vi "Camera Tester.vi"() -> ()   [LabVIEW 2024]
doc: "Use this template to build a user interface event handler design pattern. Use this pattern for dialog boxes and other user interfaces. You also can create and execute user-defined events that the VI can handle the same way as user interface events."
uses:
  camera.ctl
  camera driver.ctl
  <vilib>/event_ctls.llb/lveventtype.ctl
  Vision.lvlib
  <vilib>/Utility/error.llb/DialogType.ctl
panel:
  in  "refresh cameras":bool
  in  "Enable imaqdx":bool
  out "String":string
  in  "info tabs":enum32{"Modes", "Properties"}(tab)
  out "Available modes":string
  out "properties":string
  out "Image":T1(plugin-control)
  in  "Save Config":bool
  in  "Open Camera":bool
  out "Camera Selection":T2[](array[typedef])
  in  "Close Camera":bool
  # "Scroll to select camera. If your camera does not show up, try enabling\nimaqdx and refreshing the list."
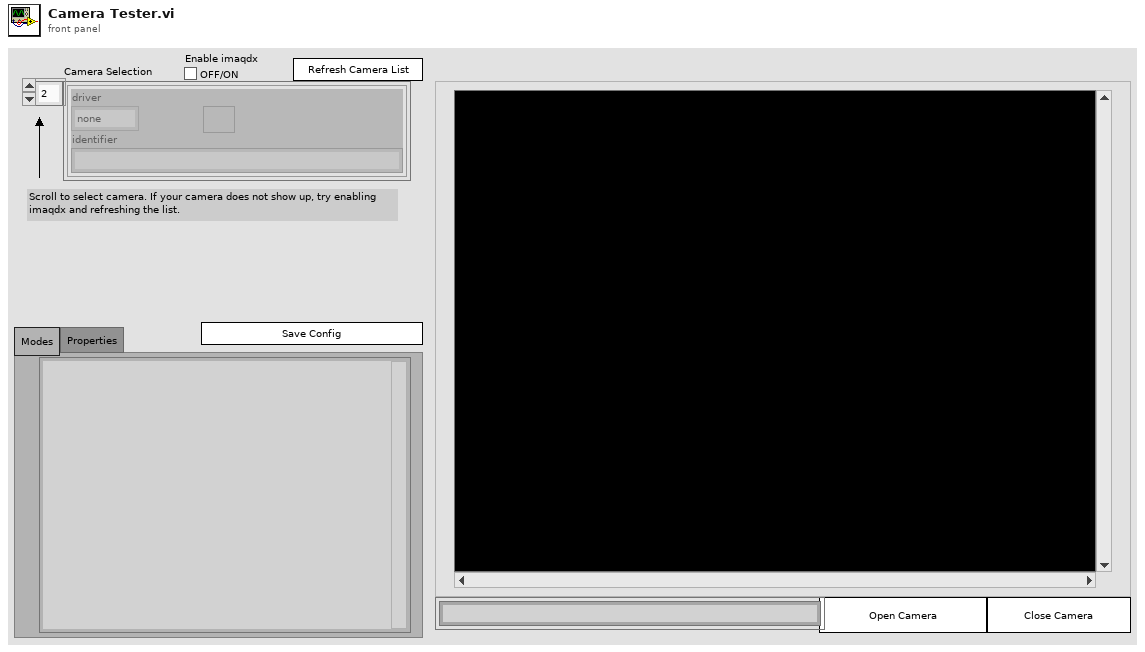
[diagram p1: front panel]
types:
  T1 = typedef "IMAQ Image.ctl" = refnum<image>
  T2 = typedef "Vision.lvlib/camera.ctl" = cluster{"camera reference":variant, "driver":T3, "identifier":string}
  T3 = typedef "Vision.lvlib/camera driver.ctl" = enum16{"none", "wmf", "imaqdx", "peak"}
  T4 = enum8{"Enabled", "Disabled", "Disabled and Grayed Out"}
  T5 = typedef "lveventtype.ctl" = enum32{"Null", "Timeout", "Annotation Menu Selection", "Annotation Menu Selection?", "App Instance Close", "App Instance Close?", "Autoscale Range Change", "Bookmark Info Change", "Cell Edit", "Cell Edit?", "Cursor Grab", "Cursor Grab?", "Cursor Menu Selection", "Cursor Menu Selection?", "Cursor Move", "Cursor Release", "Data Change", "Direction Change", "Display State Change", "Drag Ended", "Drag Enter", "Drag Leave", "Drag Over", "Drag Source Update", "Drag Starting", "Drag Starting?", "Drop", "Exec State Change", "Key Down", "Key Down?", "Key Repeat", "Key Repeat?", "Key Up", "Listbox Double Click", "Menu Activation?", "Menu Selection (App)", "Menu Selection? (App)", "Menu Selection (User)", "Mouse Down", "Mouse Down?", "Mouse Enter", "Mouse Leave", "Mouse Move", "Mouse Up", "Mouse Wheel", "NI Security User Change (App)", "Pane Size", "Panel Close", "Panel Close?", "Panel Resize", "Plot Attribute Change", "Scale Range Change", "Shortcut Menu Activation?", "Shortcut Menu Selection (App)", "Shortcut Menu Selection? (App)", "Shortcut Menu Selection (User)", "Tree Double Click", "Tree Drag", "Tree Drag?", "Tree Drop", "Tree Drop?", "Tree Item Close", "Tree Item Close?", "Tree Item Open", "Tree Item Open?", "User Event", "Value Change"}
  T6 = typedef "DialogType.ctl" = u16
  T7 = typedef "camera mode.ctl" = cluster{"id":i32, "width":i32, "height":i32, "framerate":sgl}
  T8 = cluster{"prop name":string, "value":sgl, "auto":bool}[]
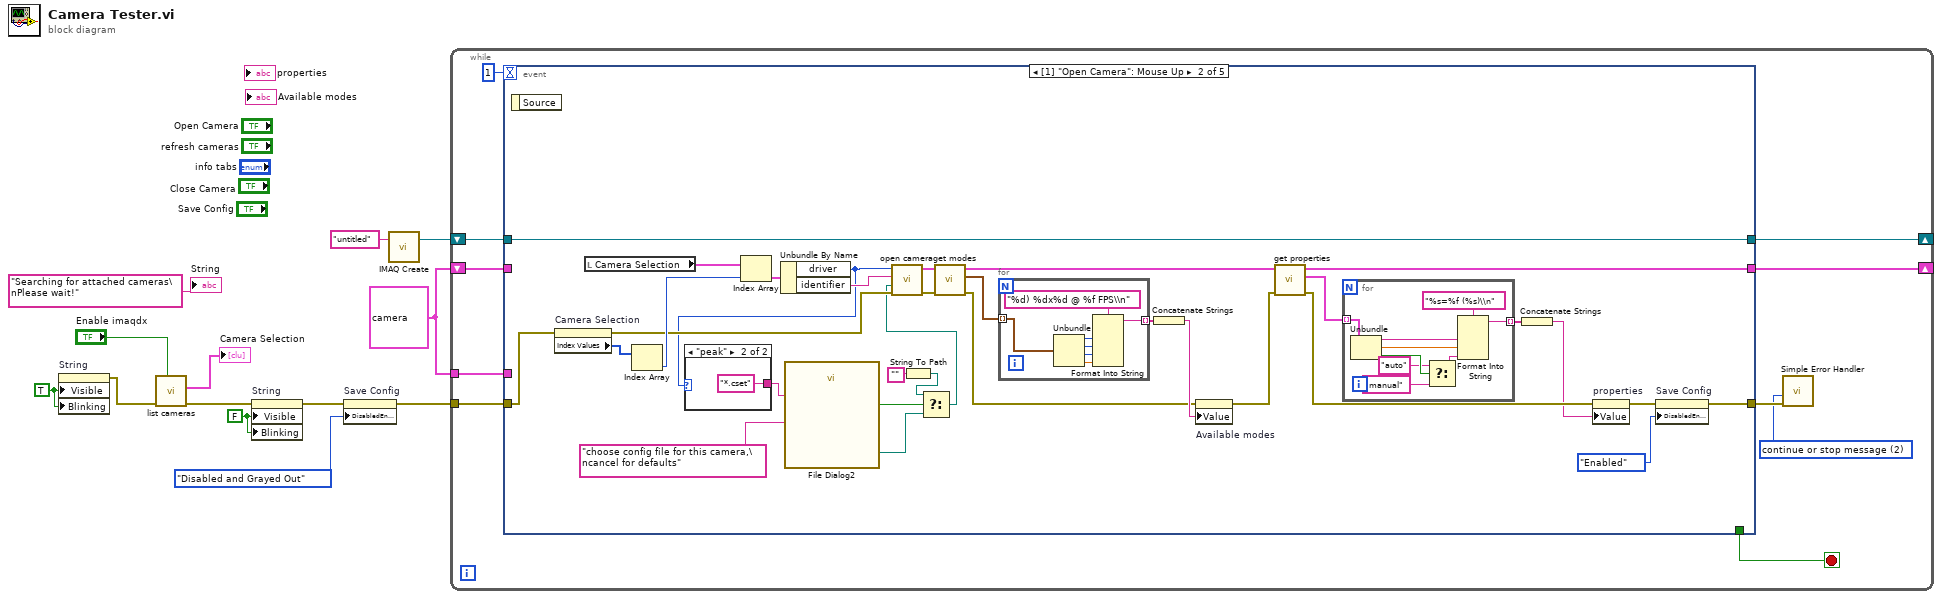
[diagram p0: block diagram]
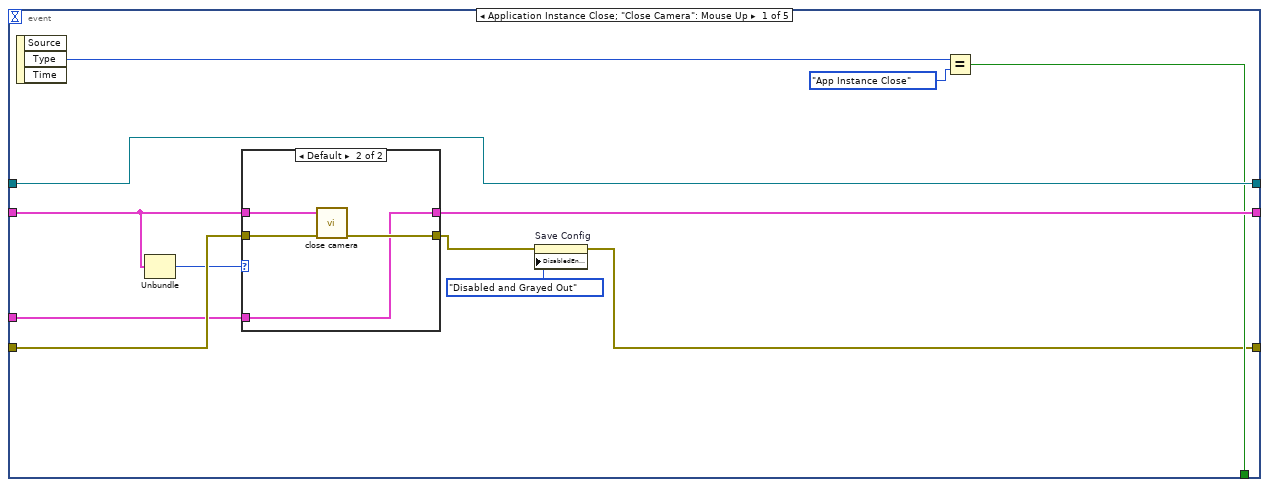
[diagram p2: hidden frame]
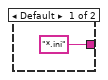
[diagram p4: hidden frame]
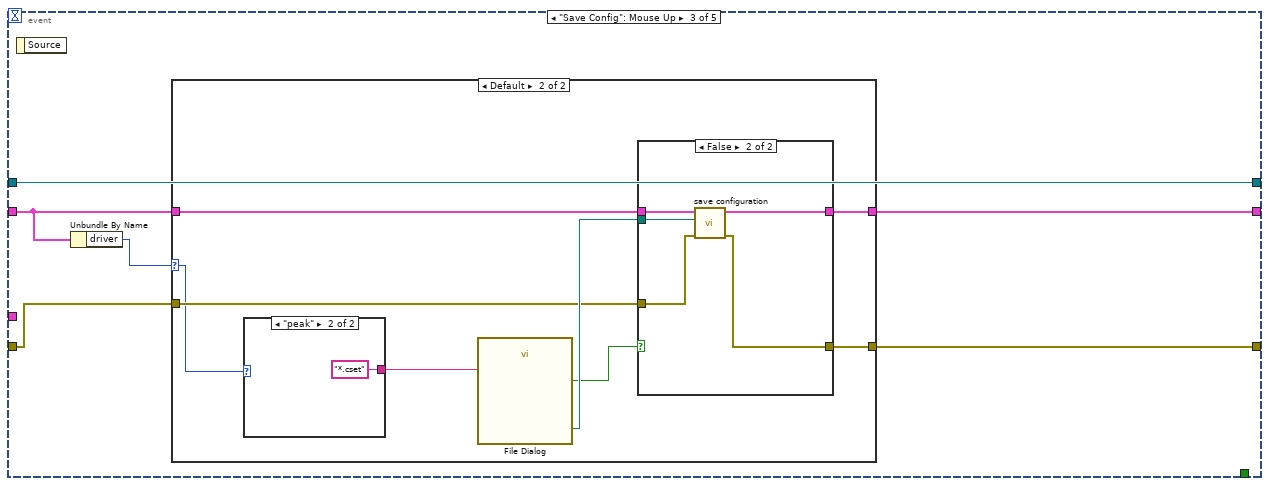
[diagram p5: hidden frame]
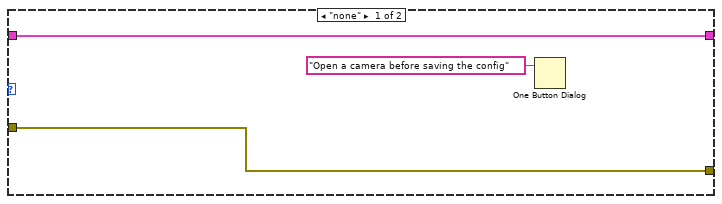
[diagram p6: hidden frame]
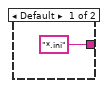
[diagram p7: hidden frame]
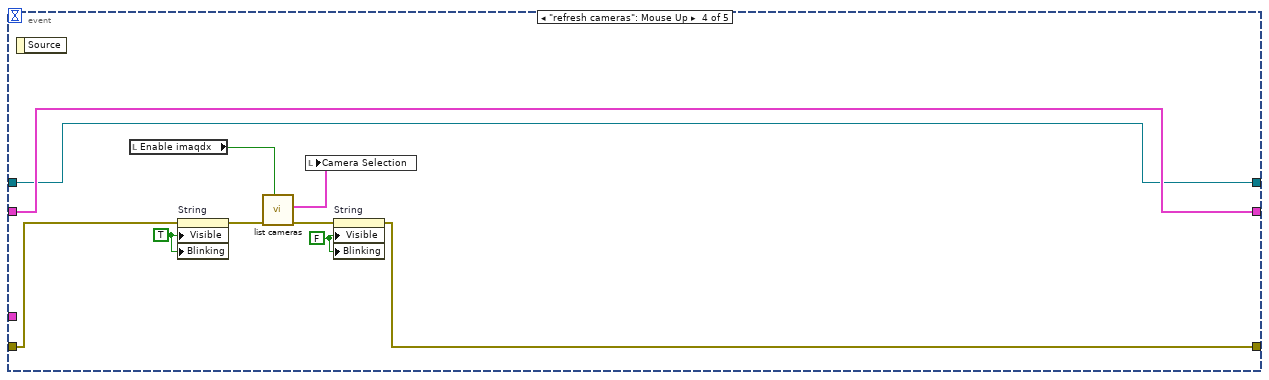
[diagram p9: hidden frame]
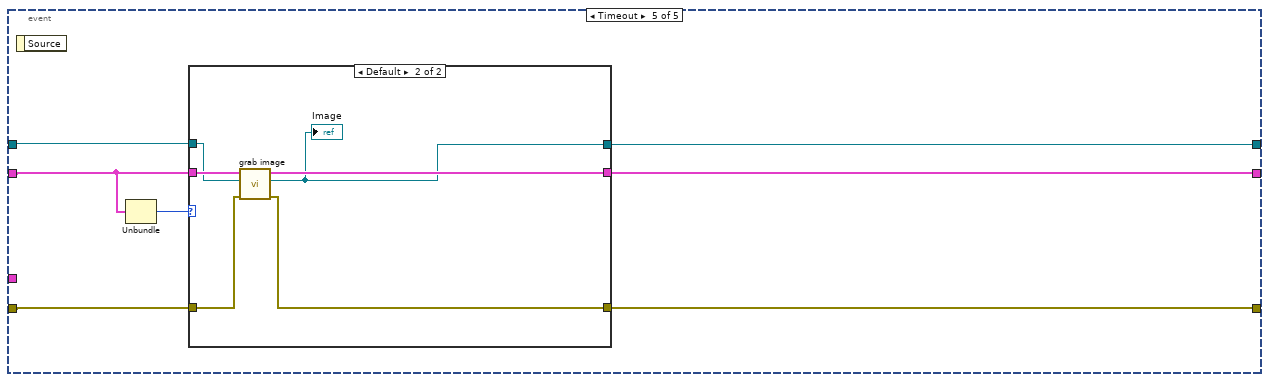
[diagram p10: hidden frame]
diagram:
  w6 = FALSE ("Visible")
  w8 = TRUE ("Visible")
  w4 = T2 {"camera reference"=variant, "driver"=enum."none", "identifier"=""} ("Camera")
  n1 = property on="String" class="Str"("Visible"=w8, "Blinking"=w8) -> (error out=w9:errorcluster)  [unwired: 2 in, 1 out]
  n2 = call "list cameras.vi"("Enable imaqdx"="Enable imaqdx", "error in (no error)"=w9) -> ("error out"=w7:errorcluster, "Cameras"=→"Camera Selection":T2[])  [unwired: 8 in]
  n3 = property on="String" class="Str"(error in=w7, "Visible"=w6, "Blinking"=w6) -> (error out=w2:errorcluster)  [unwired: 1 in, 1 out]
  n4 = property on="Save Config" class="Bool (strict)"(error in=w2, "DisabledEnum"=T4."Disabled and Grayed Out" ("Disabled")) -> (error out=w1:errorcluster)  [unwired: 1 in, 1 out]
  n5 = call "IMAQ Create"("Image Name"="untitled") -> ("New Image"=w12:T1)  [unwired: 4 in, 1 out]
  n6 = while {
    tunnel: w1 -> [w21]
    shift-right: [w19] -> _
    shift-left: w4 -> [w18]
    shift-right: [w17] -> _
    shift-left: w12 -> [w22]
    tunnel: w4 -> [w16]
    stop <- w15 stop-if-true
    w14 = T6 2 items=["no dialog", "OK message", "continue or stop message", "OK message + warnings", "continue/stop + warnings"] ("type of dialog (OK msg:1)")
    n7 = event shown="[1] \"Open Camera\": Mouse Up" {
      selector: _ -> [_ _ _ _ _]
      dyn-events: _ -> [_ _ _ _ _]
      timeout: 1 -> [_ _ _ _ _]
      tunnel: [w28 _ _ _ _] -> w15
      tunnel: w22 -> [w31 w65 w97 w118 w132]
      tunnel: w21 -> [w35 w70 w95 w127 w131]
      tunnel: [w25 w42 w96 w120 w130] -> w20
      tunnel: [w31 w65 w97 w118 w128] -> w17
      tunnel: [w32 w56 w94 w119 w129] -> w19
      tunnel: w18 -> [w34 _ w93 w119 w133]
      tunnel: w16 -> [w27 _ _ _ _]
      event Application Instance Close; "Close Camera": Mouse Up {
        n8 = event-data() -> ("Type"=w30:T5)  [unwired: 1 in, 2 out]
        n9 = Unbundle(w34) -> ("driver"=w33:T3)  [unwired: 2 out]
        n10 = case shown="Default" w33 {
          tunnel: w34 -> [w37 w41]
          tunnel: w35 -> [w36 w40]
          tunnel: [w37 w38] -> w32
          tunnel: [w36 w39] -> w26
          tunnel: w27 -> [_ w38]
          frame "none" {
          }
          frame Default {
            n11 = call "close camera.vi"("error in (no error)"=w40, "Camera"=w41) -> ("error out"=w39:errorcluster)  [unwired: 8 in, 1 out]
          }
        }
        n12 = property on="Save Config" class="Bool (strict)"(error in=w26, "DisabledEnum"=T4."Disabled and Grayed Out" ("Disabled")) -> (error out=w25:errorcluster)  [unwired: 1 in, 1 out]
        n13 = Equal?(x=w30, y=lveventtype."App Instance Close") -> (x = y?=w28:bool)
      }
      event "Open Camera": Mouse Up {
        n14 = event-data() -> ()  [unwired: 1 in, 1 out]
        n15 = property on="Camera Selection" class="Arr (strict)"(error in=w70) -> (error out=w67:errorcluster, "Index Values"=w71:u32[])  [unwired: 1 in, 1 out]
        n16 = local read "Camera Selection"() -> (w68:T2[])
        n17 = Index Array(array=w71) -> (element=w69:u32)  [unwired: 1 in]
        n18 = Index Array(array=w68, index=w69) -> (element=w73:T2)
        n19 = Unbundle By Name(w73) -> ("driver"=w46:T3, "identifier"=w72:string)
        n20 = case shown="\"peak\"" w46 {
          tunnel: ["*.ini" ("pattern label") "*.cset" ("pattern label")] -> w45
          frame Default {
          }
          frame "peak" {
          }
        }
        n21 = call "File Dialog2"("prompt"="choose config file for this camera,\ncancel for defaults", "pattern (all files)"=w45) -> ("selected path"=w50:path, "cancelled"=w51:bool)  [unwired: 10 in, 2 out]
        n22 = String To Path(string="") -> (path=w49:path)
        n23 = Select(t=w49, s=w51, f=w50) -> (s? t:f=w47:path)
        n24 = call "open camera.vi"("error in (no error)"=w67, "Camera Settings"=w47, "identifier"=w72, "driver"=w46) -> ("error out"=w63:errorcluster, "Camera"=w64:T2)  [unwired: 6 in]
        n25 = call "get modes.vi"("error in (no error)"=w63, "Camera"=w64) -> ("error out"=w59:errorcluster, "Modes"=w62:T7[], "Camera out"=w58:T2)  [unwired: 7 in]
        n26 = for {
          tunnel: w62 -> [w90] mode=indexing
          tunnel: [w85] -> w61 mode=indexing
          n27 = Unbundle(w90) -> ("id"=w89:i32, "width"=w88:i32, "height"=w87:i32, "framerate"=w86:sgl)
          n28 = Format Into String(format string="%d) %dx%d @ %f FPS\\n", w89, w88, w87, w86) -> (resulting string=w85:string)  [unwired: 2 in, 1 out]
        }
        n29 = Concatenate Strings(w61) -> (w60:string)
        n30 = property on="Available modes" class="Str"(error in=w59, "Value"=w60) -> (error out=w57:errorcluster)  [unwired: 1 in, 1 out]
        n31 = call "get properties.vi"("error in (no error)"=w57, "Camera"=w58) -> ("error out"=w54:errorcluster, "Properties"=w55:T8, "Camera out"=w56:T2)  [unwired: 7 in]
        n32 = for {
          tunnel: w55 -> [w83] mode=indexing
          tunnel: [w81] -> w53 mode=indexing
          n33 = Unbundle(w83) -> ("prop name"=w80:string, "value"=w82:sgl, "auto"=w79:bool)
          n34 = Select(t="auto", s=w79, f="manual") -> (s? t:f=w76:string)
          n35 = Format Into String(format string="%s=%f (%s)\\n", w80, w82, w76) -> (resulting string=w81:string)  [unwired: 2 in, 1 out]
        }
        n36 = Concatenate Strings(w53) -> (w52:string)
        n37 = property on="properties" class="Str"(error in=w54, "Value"=w52) -> (error out=w44:errorcluster)  [unwired: 1 in, 1 out]
        n38 = property on="Save Config" class="Bool (strict)"(error in=w44, "DisabledEnum"=T4."Enabled" ("Disabled")) -> (error out=w42:errorcluster)  [unwired: 1 in, 1 out]
      }
      event "Save Config": Mouse Up {
        n39 = event-data() -> ()  [unwired: 1 in, 1 out]
        n40 = Unbundle By Name(w93) -> ("driver"=w92:T3)
        n41 = case shown="Default" w92 {
          selector: w92 -> [_ w102]
          tunnel: [w98 w107] -> w96
          tunnel: w95 -> [w98 w106]
          tunnel: [w99 w105] -> w94
          tunnel: w93 -> [w99 w104]
          frame "none" {
            n42 = One Button Dialog(message="Open a camera before saving the config") -> ()  [unwired: 1 in, 1 out]
          }
          frame Default {
            n43 = case shown="\"peak\"" w102 {
              tunnel: ["*.ini" ("pattern label") "*.cset" ("pattern label")] -> w101
              frame Default {
              }
              frame "peak" {
              }
            }
            n44 = call "File Dialog"("pattern (all files)"=w101) -> ("selected path"=w108:path, "cancelled"=w103:bool)  [unwired: 11 in, 2 out]
            n45 = case shown="False" w103 {
              tunnel: w108 -> [_ w117]
              tunnel: [w112 w116] -> w107
              tunnel: w106 -> [w112 w115]
              tunnel: [w111 w114] -> w105
              tunnel: w104 -> [w111 w113]
              frame True {
              }
              frame False {
                n46 = call "save configuration.vi"("error in (no error)"=w115, "Path"=w117, "Camera"=w113) -> ("error out"=w116:errorcluster, "Camera out"=w114:T2)  [unwired: 7 in]
              }
            }
          }
        }
      }
      event "refresh cameras": Mouse Up {
        w121 = FALSE ("Visible")
        w122 = TRUE ("Visible")
        n47 = event-data() -> ()  [unwired: 1 in, 1 out]
        n48 = local read "Enable imaqdx"() -> (w125:bool)
        n49 = property on="String" class="Str"(error in=w127, "Visible"=w122, "Blinking"=w122) -> (error out=w126:errorcluster)  [unwired: 1 in, 1 out]
        n50 = call "list cameras.vi"("Enable imaqdx"=w125, "error in (no error)"=w126) -> ("error out"=w123:errorcluster, "Cameras"=w124:T2[])  [unwired: 8 in]
        n51 = local write "Camera Selection"(w124) -> ()
        n52 = property on="String" class="Str"(error in=w123, "Visible"=w121, "Blinking"=w121) -> (error out=w120:errorcluster)  [unwired: 1 in, 1 out]
      }
      event Timeout {
        n53 = event-data() -> ()  [unwired: 1 in, 1 out]
        n54 = Unbundle(w133) -> ("driver"=w134:T3)  [unwired: 2 out]
        n55 = case shown="Default" w134 {
          tunnel: w133 -> [w135 w143]
          tunnel: w132 -> [w137 w142]
          tunnel: [w135 w141] -> w129
          tunnel: w131 -> [w136 w140]
          tunnel: [w136 w139] -> w130
          tunnel: [w137 w138] -> w128
          frame "none" {
          }
          frame Default {
            n56 = call "grab image.vi"("error in (no error)"=w140, "Image In"=w142, "Camera"=w143) -> ("error out"=w139:errorcluster, "Image Out"=w138:T1, "Camera out"=w141:T2)  [unwired: 6 in]
            "Image" <- w138
          }
        }
      }
    }
    n57 = call <vilib>:"Simple Error Handler.vi"("type of dialog (OK msg:1)"=w14, "error in (no error)"=w20) -> ()  [unwired: 3 in, 5 out]
  }
  "String" <- "Searching for attached cameras\nPlease wait!" ("String")
